vi "nPoint_id_slew_OL_FIFO_input.vi"() -> ()   [LabVIEW 2017]
uses:
  <vilib>/rvi/Emulation/niFpgaGetClockAttributes.vi
  <vilib>/rvi/Emulation/niFpgaSctlEmulationGetInTimedLoop.vi
  <vilib>/rvi/Emulation/niFpgaEmulationReportErrorSimple.vi
  <vilib>/rvi/eio/common/nirviEmuTemplateMethod_errors.vi
  <vilib>/rvi/interface/RandomDataEmulation/niFpgaRandomDataHandleErrors.vi
  <vilib>/rvi/Emulation/niFpgaCriticalErrorInLSC.vi
  <vilib>/eio/EIONode/EIONode.xnode
  <vilib>/rvi/DataTransferAndStorage/Container/XNode/niFpgaContainer.xnode
  <vilib>/rvi/interface/RandomDataEmulation/nirviRandomDataFpgaReadWriteTemplate.vi
panel:
  out "Timed Out?":bool
  out "YK TO":bool
  out "Unstable Traj":bool
  out "Loop Done":bool
  in  "Abort":bool=TRUE
  in  "ymax":sgl=4.0 format="%#_13g"
  in  "TsTicks":i16
  out "Loop Ticks (benchmark)":i16
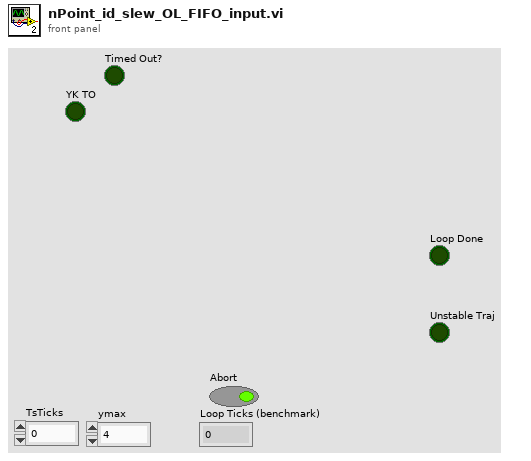
[diagram p1: front panel]
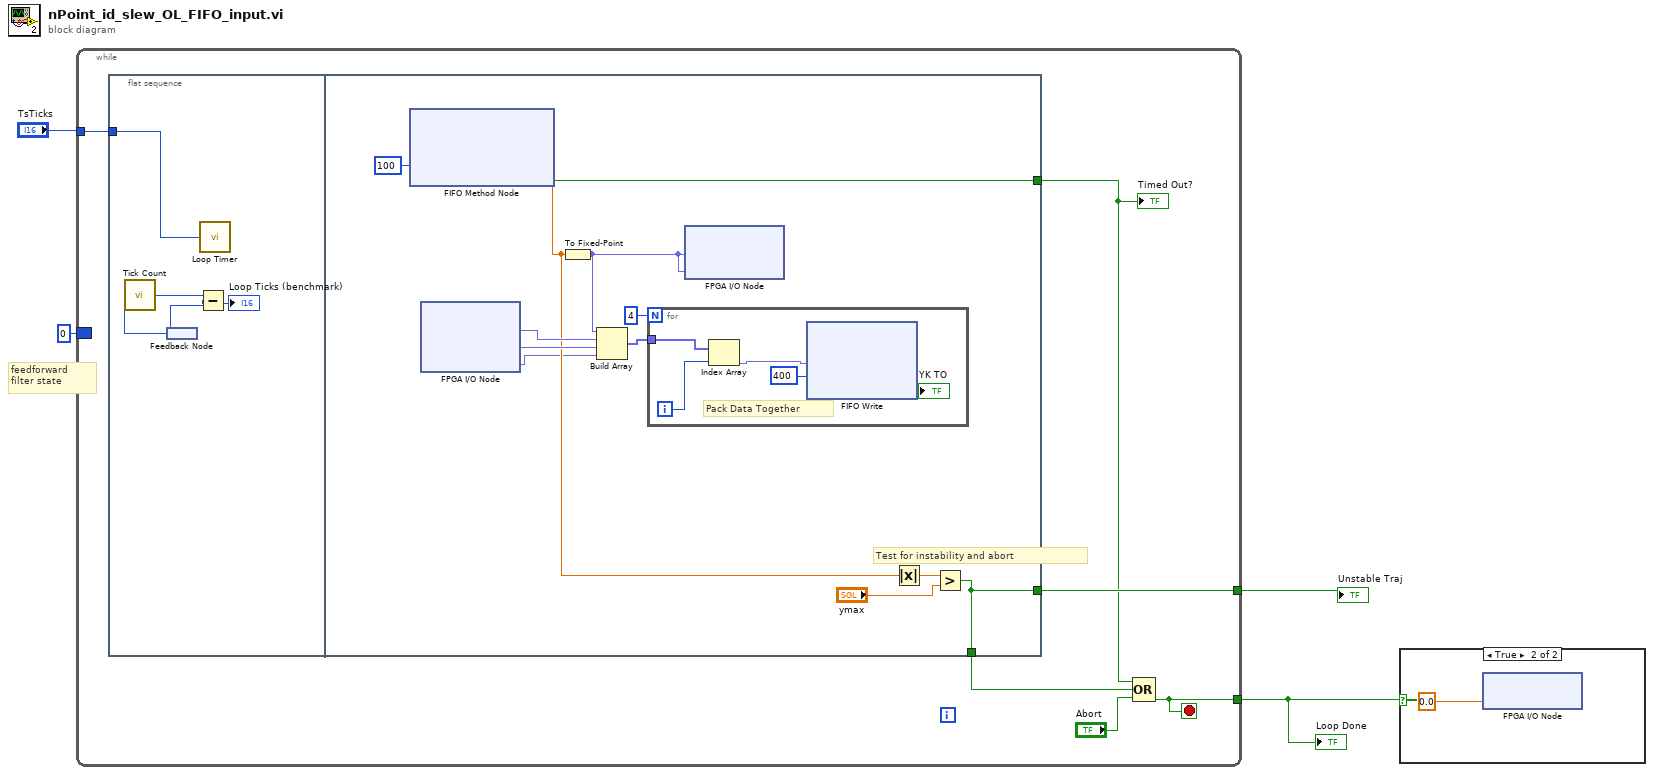
[diagram p0: block diagram]
diagram:
  # "feedforward\nfilter state"
  n1 = while {
    border: i16 0 -> [_]
    tunnel: "TsTicks" -> [w10]
    tunnel: [w7] -> w1
    tunnel: [w9] -> w3
    stop <- w7 stop-if-true
    n2 = flat-sequence {
      tunnel: w10 -> [w11]
      tunnel: [w23] -> w8
      tunnel: [w23] -> w9
      tunnel: [w17] -> w5
      frame #0 {
        n3 = call "Tick Count"() -> ("Tick Count(Ticks)"=w12:u32)
        n4 = feedback #1() -> (w13:u32)
        n5 = feedback-in #1(w12) -> ()
        n6 = Subtract(x=w12, y=w13) -> (x-y=→"Loop Ticks (benchmark)":u32)
        n7 = call "Loop Timer"("Count(Ticks)"=w11) -> ()  [unwired: 1 out]
      }
      frame #1 {
        # "Test for instability and abort"
        n8 = xnode ("FIFO Method Node")("Timeout"=100) -> ("Element"=w19:sgl, "Timed Out?"=w17:bool)  [unwired: 1 in, 1 out]
        n9 = xnode "FPGA I/O Node"() -> ("Mod2/AI0"=w22:fxp<+/-,24,5>, "Mod2/AI1"=w20:fxp<+/-,24,5>, "Mod2/AI2"=w16:fxp<+/-,24,5>)  [unwired: 3 in, 3 out]
        n10 = To Fixed-Point(number=w19) -> (fixed-point=w15:fxp<+/-,32,6>)  [unwired: 1 in]
        n11 = Build Array(w15, w22, w20, w16) -> (w24:fxp<+/-,32,6>[])
        n12 = for {
          N: 4 -> [_]
          tunnel: w24 -> [w29]
          i -> [w30]
          # "Pack Data Together"
          n13 = Index Array(array=w29, index=w30) -> (element=w27:fxp<+/-,32,6>)
          n14 = xnode ("FIFO Write")("Element"=w27, "Timeout"=i16 400) -> ("Timed Out?"=→"YK TO":bool)  [unwired: 1 in, 1 out]
        }
        n15 = xnode "FPGA I/O Node"("Mod1/AO0"=w15, "Mod1/AO1"=w15) -> ()  [unwired: 2 in, 2 out]
        n16 = Absolute Value(x=w19) -> (abs(x)=w26:sgl)
        n17 = Greater?(x=w26, y="ymax") -> (0:w23:bool)
      }
    }
    n18 = Compound Arithmetic op=OR(w5, w8, "Abort") -> (w7:bool)
    "Timed Out?" <- w5
  }
  "Loop Done" <- w1
  "Unstable Traj" <- w3
  n19 = case shown="True" w1 {
    frame False {
    }
    frame True {
      n20 = xnode "FPGA I/O Node"("Mod1/AO0"=sgl 0.0) -> ()  [unwired: 1 in, 1 out]
    }
  }
